vi "Overwrite Project Data.vi"(8 "error in (no error)":errorcluster, 10 "Project Data":refnum<class "Project Data.lvclass">, 11 "Project Data ref in":refnum<data-value>) -> (0 "error out":errorcluster, 3 "Project Data ref out":refnum<data-value>)   [LabVIEW 2013, in "SET Project Editor.lvlib" / "New Project Wizard.lvclass"]
uses:
  New Project Wizard.lvclass
  SET Project Data/Project Data Class/Project Data.lvclass
  SET Project Data/Resource Data Class/Resource Data.lvclass
  SET Project Data/Project Data Class/Write Resource Data ref.vi
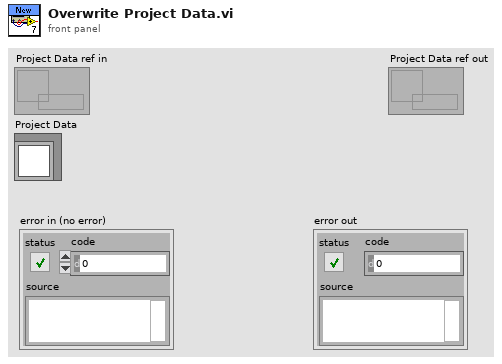
[diagram p1: front panel]
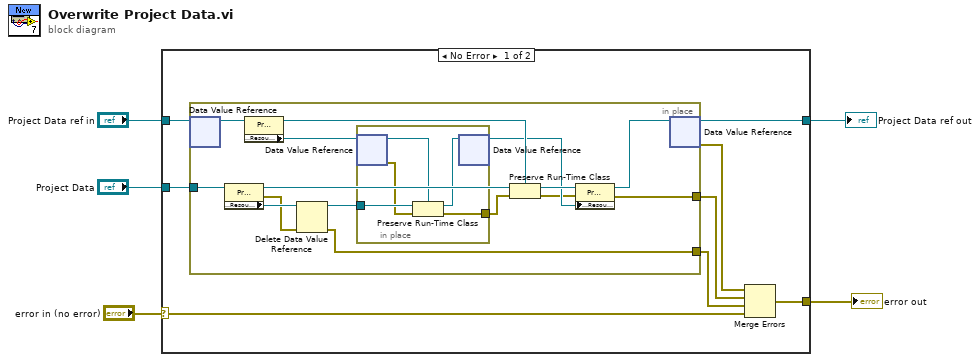
[diagram p0: block diagram]
diagram:
  n1 = case shown="No Error" "error in (no error)" {
    selector: "error in (no error)" -> [w7 w34]
    tunnel: "Project Data ref in" -> [w13 w35]
    tunnel: [w12 w35] -> w4
    tunnel: "Project Data" -> [w11 _]
    tunnel: [w6 w34] -> w1
    frame No Error {
      n2 = in-place {
        in-place-border: w11 -> [w28]
        in-place-border: [w16] -> w9
        in-place-border: [w14] -> w8
        n3 = in-place-dvr #1(w13) -> (w26:refnum<class "Project Data.lvclass">)  [unwired: 1 out]
        n4 = property class="Project Data.lvclass"(reference=w28) -> (reference out=w24:refnum<class "Project Data.lvclass">, error out=w15:errorcluster, "Properties:Resource Data ref"=w27:refnum<data-value>)  [unwired: 1 in]
        n5 = property class="Project Data.lvclass"(reference=w26) -> (reference out=w25:refnum<class "Project Data.lvclass">, "Properties:Resource Data ref"=w23:refnum<data-value>)  [unwired: 1 in, 1 out]
        n6 = Delete Data Value Reference(data value reference=w27, error in=w15) -> (data value=w22:refnum<class "Resource Data.lvclass">, error out=w14:errorcluster)
        n7 = in-place {
          in-place-border: w22 -> [w32]
          in-place-border: [w29] -> w18
          n8 = in-place-dvr #2(w23) -> (w33:refnum<class "Resource Data.lvclass">, w30:errorcluster)
          n9 = Preserve Run-Time Class(object in=w32, error in=w30, 2:w33) -> (object out=w31:refnum<class "Resource Data.lvclass">, error out=w29:errorcluster)
          n10 = in-place-dvr #2(w31) -> (w20:refnum<data-value>)  [unwired: 1 out]
        }
        n11 = Preserve Run-Time Class(object in=w24, error in=w18, 2:w25) -> (object out=w21:refnum<class "Project Data.lvclass">, error out=w17:errorcluster)
        n12 = property class="Project Data.lvclass"(reference=w21, error in=w17, "Properties:Resource Data ref"=w20) -> (reference out=w19:refnum<class "Project Data.lvclass">, error out=w16:errorcluster)
        n13 = in-place-dvr #1(w19) -> (w12:refnum<data-value>, w10:errorcluster)
      }
      n14 = Merge Errors(w10, w9, w8, w7) -> (w6:errorcluster)
    }
    frame Error {
    }
  }
  "Project Data ref out" <- w4
  "error out" <- w1
